vi "Read Parameters of measurement.vi"(8 "error in (no error)":errorcluster caption="entrée d'erreur (pas d'erreur)", 11 "Control-Client en entrée":refnum<class "Control-Client.lvclass">) -> (0 "error out":errorcluster caption="sortie d'erreur", 2 "cluster d'entrée":T1={"ODmin"=-0.35, "ODmax"=0.35, "Aq contol"=enum."fixed", "Wavelength_fix_index"=640, "WCM_limits"={"WCM_min"=0.0, "WCM_max"=0.0, "WCM_value"=0.0}, "WCM_corrections"=FALSE, "#cycles max"=5}, 3 "Control-Client en sortie":refnum<class "Control-Client.lvclass">)   [LabVIEW 2019, in "Control-Client.lvclass"]
uses:
  Control-Client.lvclass
  dependecies/ControlsVIs/Clusters-def/Parameters_measurement_def.ctl
  Control-Client.lvclass/Control-Client.ctl
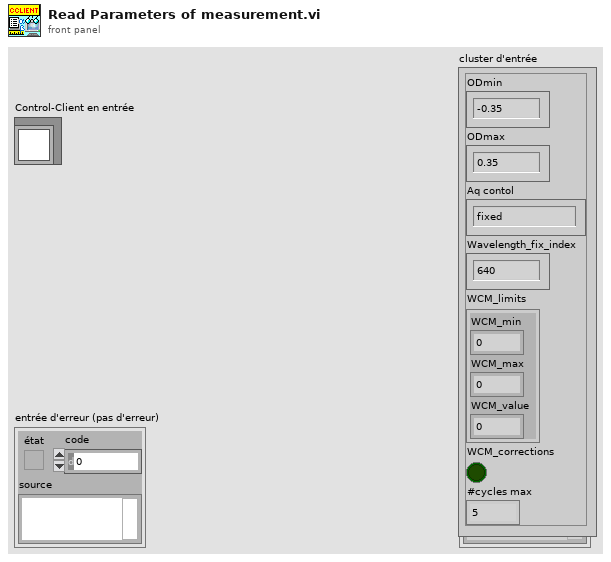
[diagram p1: front panel]
types:
  T1 = typedef "Parameters_measurement_def.ctl" = cluster{"ODmin":dbl, "ODmax":dbl, "Aq contol":enum32{"fixed", "automatic", "fixed-auto"}, "Wavelength_fix_index":i32, "WCM_limits":cluster{"WCM_min":dbl, "WCM_max":dbl, "WCM_value":dbl}, "WCM_corrections":bool, "#cycles max":i32}
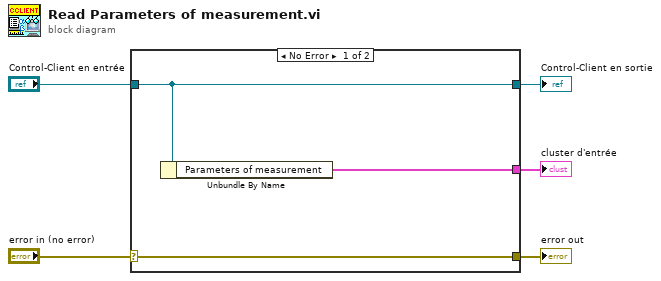
[diagram p0: block diagram]
diagram:
  n1 = case shown="No Error" "error in (no error)" {
    selector: "error in (no error)" -> [w8 w9]
    tunnel: [w8 w9] -> w4
    tunnel: [w7 w10] -> w2
    tunnel: "Control-Client en entrée" -> [w7 w10]
    tunnel: [w6 _] -> w1
    frame No Error {
      n2 = Unbundle By Name(w7) -> ("Parameters of measurement"=w6:T1)
    }
    frame Error {
    }
  }
  "error out" <- w4
  "Control-Client en sortie" <- w2
  "cluster d'entrée" <- w1
